vi "Write_TriggerStateChange.vi"(8 "error in (no error)":errorcluster, 10 "Trigger":enum16{"Off", "On"}(ring), 11 "Multiplexer_Opmux in":refnum<class "Multiplexer_Opmux.lvclass">) -> (0 "error out":errorcluster, 3 "Multiplexer_Opmux out":refnum<class "Multiplexer_Opmux.lvclass">)   [LabVIEW 2014, in "Multiplexer_Opmux.lvclass"]
uses:
  Multiplexer_Opmux.lvclass
  Multiplexer_Opmux.lvclass/Multiplexer_Opmux.ctl
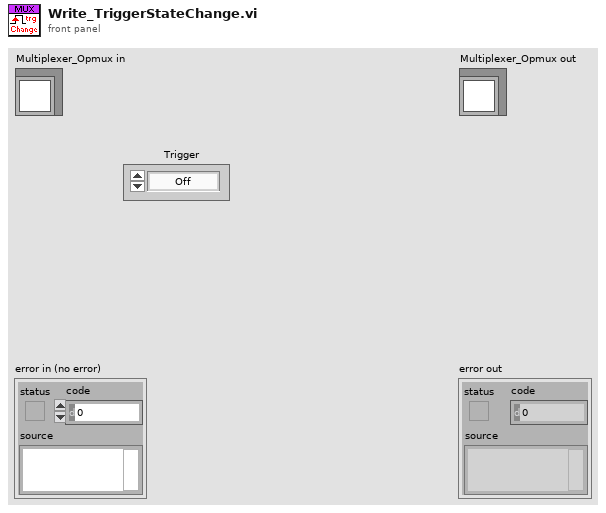
[diagram p1: front panel]
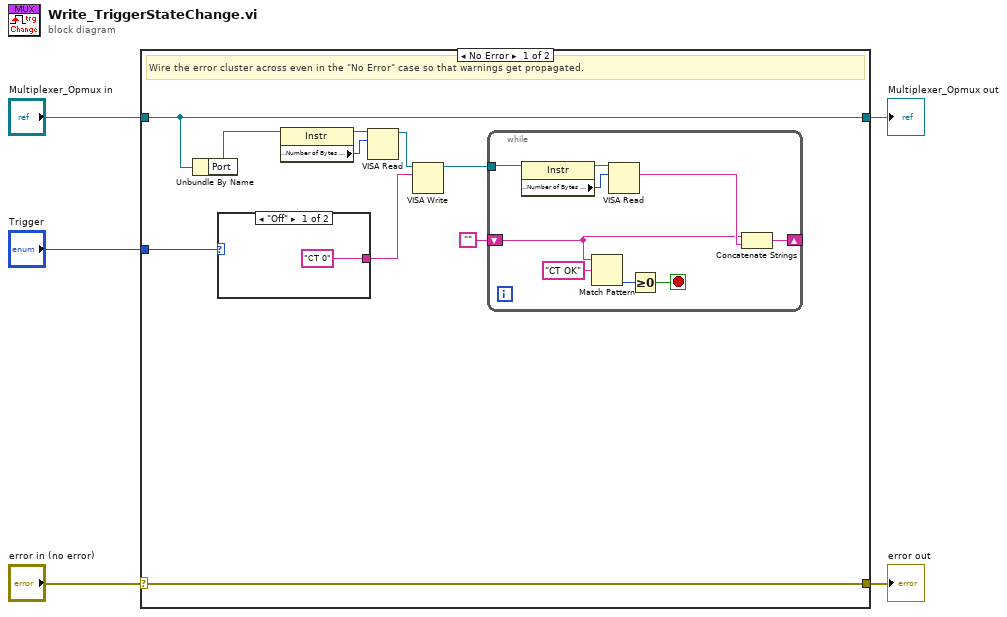
[diagram p0: block diagram]
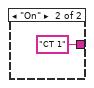
[diagram p2: hidden frame]
diagram:
  n1 = case shown="No Error" "error in (no error)" {
    selector: "error in (no error)" -> [w14 w28]
    tunnel: [w14 w28] -> w4
    tunnel: [w15 w27] -> w2
    tunnel: "Multiplexer_Opmux in" -> [w15 w27]
    tunnel: "Trigger" -> [w7 _]
    frame No Error {
      # "Wire the error cluster across even in the \"No Error\" case so that warnings get propagated."
      n2 = Unbundle By Name(w15) -> ("Port"=w9:refnum<visa-resource-name>)
      n3 = case shown="\"Off\"" w7 {
        tunnel: ["CT 0" "CT 1"] -> w6
        frame "Off" {
        }
        frame "On" {
        }
      }
      n4 = property class="Instr"(reference=w9) -> (reference out=w11:refnum<visa-resource-name>, "Serial Settings:Number of Bytes at Serial Port"=w10:u32)  [unwired: 1 in, 1 out]
      n5 = VISA Read(VISA resource name=w11, byte count=w10) -> (VISA resource name out=w8:refnum<visa-resource-name>)  [unwired: 1 in, 3 out]
      n6 = VISA Write(VISA resource name=w8, write buffer=w6) -> (VISA resource name out=w12:refnum<visa-resource-name>)  [unwired: 1 in, 2 out]
      n7 = while {
        shift-right: [w23] -> _
        shift-left: "" -> [w20]
        tunnel: w12 -> [w25]
        stop <- w18 stop-if-true
        n8 = property class="Instr"(reference=w25) -> (reference out=w26:refnum<visa-resource-name>, "Serial Settings:Number of Bytes at Serial Port"=w24:u32)  [unwired: 1 in, 1 out]
        n9 = Match Pattern(string=w20, regular expression="CT OK") -> (offset past match=w19:i32)  [unwired: 1 in, 3 out]
        n10 = VISA Read(VISA resource name=w26, byte count=w24) -> (read buffer=w22:string)  [unwired: 1 in, 3 out]
        n11 = Greater Or Equal To 0?(x=w19) -> (x >= 0?=w18:bool)
        n12 = Concatenate Strings(w20, w22) -> (w23:string)
      }
    }
    frame Error {
    }
  }
  "error out" <- w4
  "Multiplexer_Opmux out" <- w2
